vi "visionTesting.vi"() -> ()   [LabVIEW 2013]
uses:
  Program Files (x86)/National Instruments/LabVIEW 2013/examples/FRC/Vision/2014 Target Detection/TargetType.ctl
  <vilib>/Rock Robotics/WPI/Camera/WPI_CameraSettings Read MJPG.ctl
  <vilib>/Rock Robotics/WPI/Camera/WPI_CameraImageSize.ctl
panel:
  in  "stop":bool
  in  "Camera Address":string="192.168.0.90"
  out "Image":T1(plugin-control)
  in  "Camera Settings":T2={"fps"=15, "compression"=5, "Image Size"=enum."320x240"}
  in  "Color Components":T4={"Hue"={80.65384674072266, 112.65384674072266}, "Sat"={49.712730407714844, 255.0}, "Val"={73.74692153930664, 173.4838523864746}}
  out "output color":T5
  out "Target Info":T7(array[cluster])
  in  "error in (no error)":errorcluster
  out "Error":bool
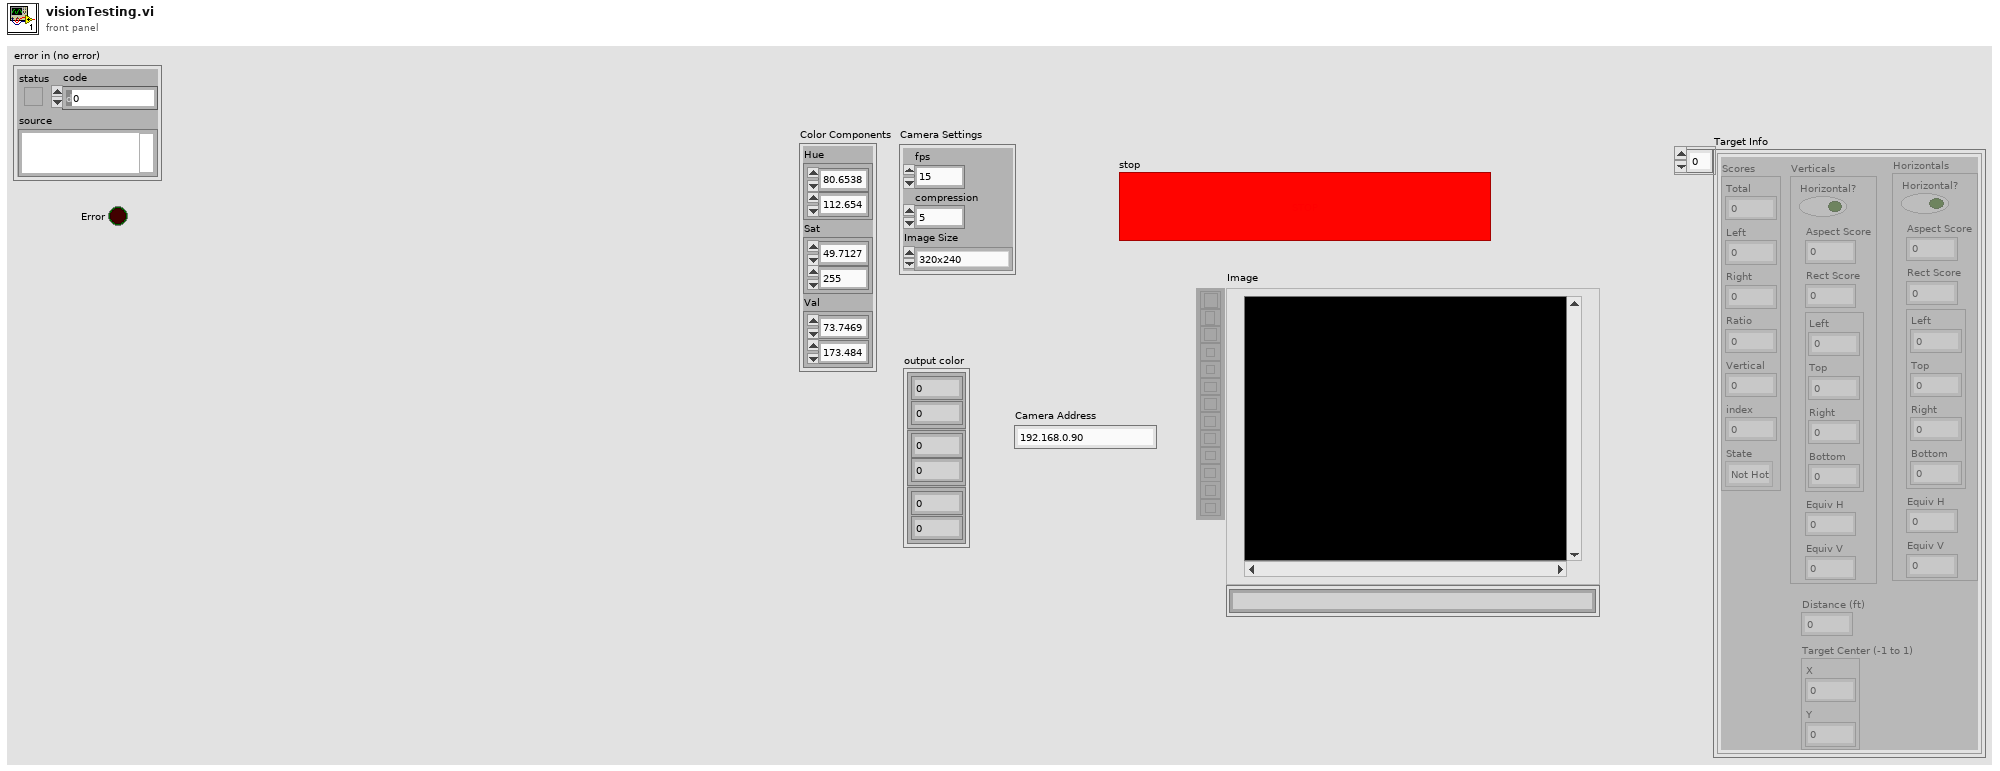
[diagram p1: front panel]
types:
  T1 = typedef "IMAQ Image.ctl" = refnum<image>
  T2 = typedef "WPI_CameraSettings Read MJPG.ctl" = cluster{"fps":i32, "compression":i32, "Image Size":T3}
  T3 = typedef "WPI_CameraImageSize.ctl" = enum16{"640x480", "320x240", "160x120"}
  T4 = cluster{"Hue":cluster{dbl, dbl}, "Sat":cluster{dbl, dbl}, "Val":cluster{dbl, dbl}}
  T5 = cluster{cluster{dbl, dbl}, cluster{dbl, dbl}, cluster{dbl, dbl}}
  T6 = typedef "TargetType.ctl" = enum16{"Not Hot", "Hot"}
  T7 = cluster{"Scores":cluster{"Total":dbl, "Left":dbl, "Right":dbl, "Ratio":dbl, "Vertical":dbl, "index":i32, "State":T6}, "Verticals":cluster{"Horizontal?":bool, "Aspect Score":dbl, "Rect Score":dbl, cluster{"Left":dbl, "Top":dbl, "Right":dbl, "Bottom":dbl}, "Equiv H":dbl, "Equiv V":dbl}, "Horizontals":cluster{"Horizontal?":bool, "Aspect Score":dbl, "Rect Score":dbl, cluster{"Left":dbl, "Top":dbl, "Right":dbl, "Bottom":dbl}, "Equiv H":dbl, "Equiv V":dbl}, "Distance (ft)":dbl, "Target Center (-1 to 1)":cluster{"X":dbl, "Y":dbl}}[]
  T8 = typedef "Image Type" = u32
  T9 = cluster{"Horizontal":bool, "Aspect Score":dbl, "Rect Score":dbl, cluster{"Left":dbl, "Top":dbl, "Right":dbl, "Bottom":dbl}, "Equiv H":dbl, "Equiv V":dbl}[]
  T10 = cluster{"Scores":cluster{"Total":dbl, "Left":dbl, "Right":dbl, "Ratio":dbl, "Vertical":dbl, "index":i32, "State":T6}, "Verticals":cluster{"Horizontal?":bool, "Aspect Score":dbl, "Rect Score":dbl, cluster{"Left":dbl, "Top":dbl, "Right":dbl, "Bottom":dbl}, "Equiv H":dbl, "Equiv V":dbl}, "Horizontals":cluster{"Horizontal?":bool, "Aspect Score":dbl, "Rect Score":dbl, cluster{"Left":dbl, "Top":dbl, "Right":dbl, "Bottom":dbl}, "Equiv H":dbl, "Equiv V":dbl}, "Validated":bool}[]
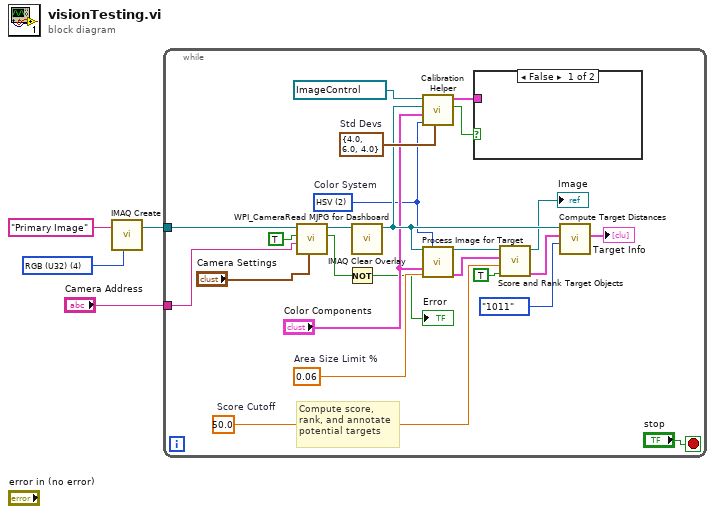
[diagram p0: block diagram]
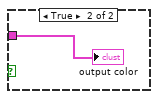
[diagram p2: hidden frame]
diagram:
  w4 = T8 4 items=["Grayscale (U8)", "Grayscale (I16)", "Grayscale (SGL)", "Complex (CSG)", "RGB (U32)", "HSL (U32)", "RGB (U64)"] ("Image Type")
  n1 = call "IMAQ Create"("Image Name"="Primary Image", "Image Type"=w4) -> ("New Image"=w2:T1)  [unwired: 2 in, 2 out]
  n2 = while {
    tunnel: w2 -> [w5]
    tunnel: "Camera Address" -> [w7]
    stop <- "stop" stop-if-true
    w28 = cluster{"Hue":dbl, "Sat":dbl, "Val":dbl} {"Hue"=4.0, "Sat"=6.0, "Val"=4.0}  # Std Devs
    w27 = 50.0  # Score Cutoff
    w26 = 0.06  # Area Size Limit %
    w16 = u16 2 items=["RGB", "HSL", "HSV", "HSI"]  # Color System
    # "Compute score,\nrank, and annotate\npotential targets"
    n3 = call <vilib>:"WPI_CameraRead MJPG for Dashboard.vi"("Camera Settings"="Camera Settings", "Camera IP"=w7, "Enable"=TRUE, "Refnum in"=w5) -> ("Active"=w23:bool, "Refnum out"=w11:T1)  [unwired: 4 in, 2 out]
    n4 = Not(x=w23) -> (.not. x?=→"Error":bool)
    n5 = call "IMAQ Clear Overlay"("Image"=w11) -> ("Image Out"=w20:T1)  [unwired: 9 in, 1 out]
    n6 = call "Calibration Helper.vi"("Std Devs"=w28, "Color Mode"=w16, "Color Components"="Color Components", "Image"=w20, "Image Ctl Refnum"=refnum<vi> refnum ("Image")) -> ("Changed"=w19:bool, "output color"=w17:T5)  [unwired: 5 in]
    n7 = call "Process Image for Target.vi"("Src Image"=w20, "Color Mode"=w16, "Color Components"="Color Components", "Area Cutoff %"=w26) -> ("Src Image Out"=w13:T1, "Particles"=w14:T9)  [unwired: 9 in, 1 out]
    n8 = case shown="False" w19 {
      tunnel: w17 -> [_ w29]
      frame False {
      }
      frame True {
        "output color" <- w29
      }
    }
    n9 = call "Score and Rank Target Objects.vi"("Annotate"=TRUE, "Score Limit"=w27, "Particles"=w14, "Image in"=w13) -> ("Target Info"=w15:T10, "Annotated Image"=→"Image":T1)  [unwired: 6 in]
    n10 = call "Compute Target Distances.vi"("Camera Type"=enum16{"206", "1011", "1013"}."1011", "Target Info"=w15, "Image in"=w20) -> ("Target Info"=→"Target Info":T7)  [unwired: 6 in, 2 out]
  }
